vi "Measurement UI.vi"() -> ()   [LabVIEW 2021, in "audio_intermodulationDistortionMeasurement.lvlib"]
uses:
  audio_intermodulationDistortionMeasurement.lvlib
panel:
  in  "Meas Graph":T1(tab)
  out "FreqDomainGraph":cluster{"x0":dbl, "dx":dbl, "magnitude":dbl[]}(graph) caption="AC"
  out "TimeDomainGraph":waveform(dbl)(graph) caption="AC"
  out "IMD":dbl
  out "f0":dbl
  out "df":dbl
  out "Freq Domain":dbl[](array[numeric])
  out "dt":dbl
  out "Time Domain":dbl[](array[numeric])
  in  "Analog Source Resource Name":string
  out "Meas Table":string[][](table)
  out "Calculated sample rate":dbl caption="SAMPLE RATE" format="%#_6pHz"
  in  "Custom High Frequency":dbl=15000.0 caption="CUSTOM HIGH FREQUENCY" format="%_2pHz"
  in  "Custom Low Frequency":dbl=14000.0 caption="CUSTOM LOW FREQUENCY" format="%#_2pHz"
  in  "MeasSettingsOptions":i32(listbox)=-1
  in  "MeasSettings":bool
  in  "Protocol settings":string="Protocol settings"
  in  "Measurement Settings":string="Analog source "
  in  "Bit Clock Rate":u32=12288000 caption="CLOCK RATE" format="%.4pHz"
  in  "Input range":dbl=2.825 caption="INPUT RANGE" format="%#_gV"
  in  "Data Latch at SCK Cycle":u8 caption="LATCH DELAY" format="%.0fs"
  in  "Number of Words":i32=19200 caption="NUMBER OF WORDS"
  in  "Protocol Source Resource Name":string="7821\\PCMi 0" caption="RESOURCE NAME"
  in  "Amplitude":dbl=-1.0 caption="AMPLITUDE" format="%#_gdB"
  in  "IMD Standard":T2(ring) caption="IMD STANDARD"
  in  "DSGResourceName":tag="PXI1Slot3/ao0" caption="RESOURCE NAME"
  in  "Custom Amplitude Ratio":dbl=1.0 caption="CUSTOM AMPLITUDE RATIO" format="%.1f"
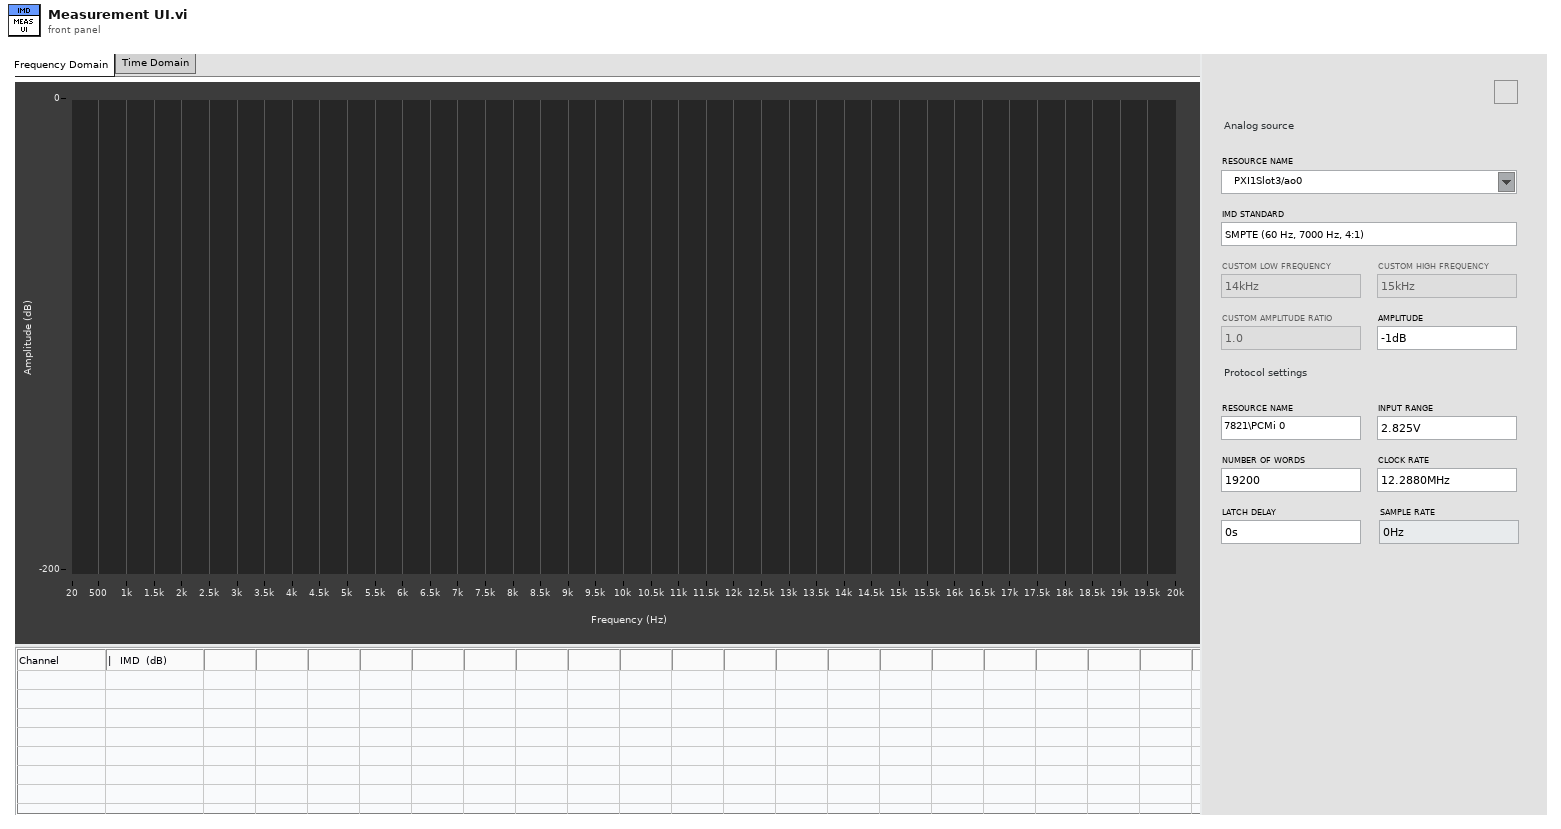
[diagram p1: front panel]
types:
  T1 = enum32{"Frequency Domain", "Time Domain", "Hidden"}
  T2 = enum16{"SMPTE (60 Hz, 7000 Hz, 4:1)", "DIN (250 Hz, 8000 Hz, 4:1)", "CCIF (11 kHz, 12 kHz, 1:1)", "CCIF (19 kHz, 20 kHz, 1:1)", "Custom"}
  T3 = enum16{"open", "replace", "create", "open or create", "replace or create", "replace or create with confirmation"}
  T4 = enum8{"Enabled", "Disabled", "Disabled and Grayed Out"}
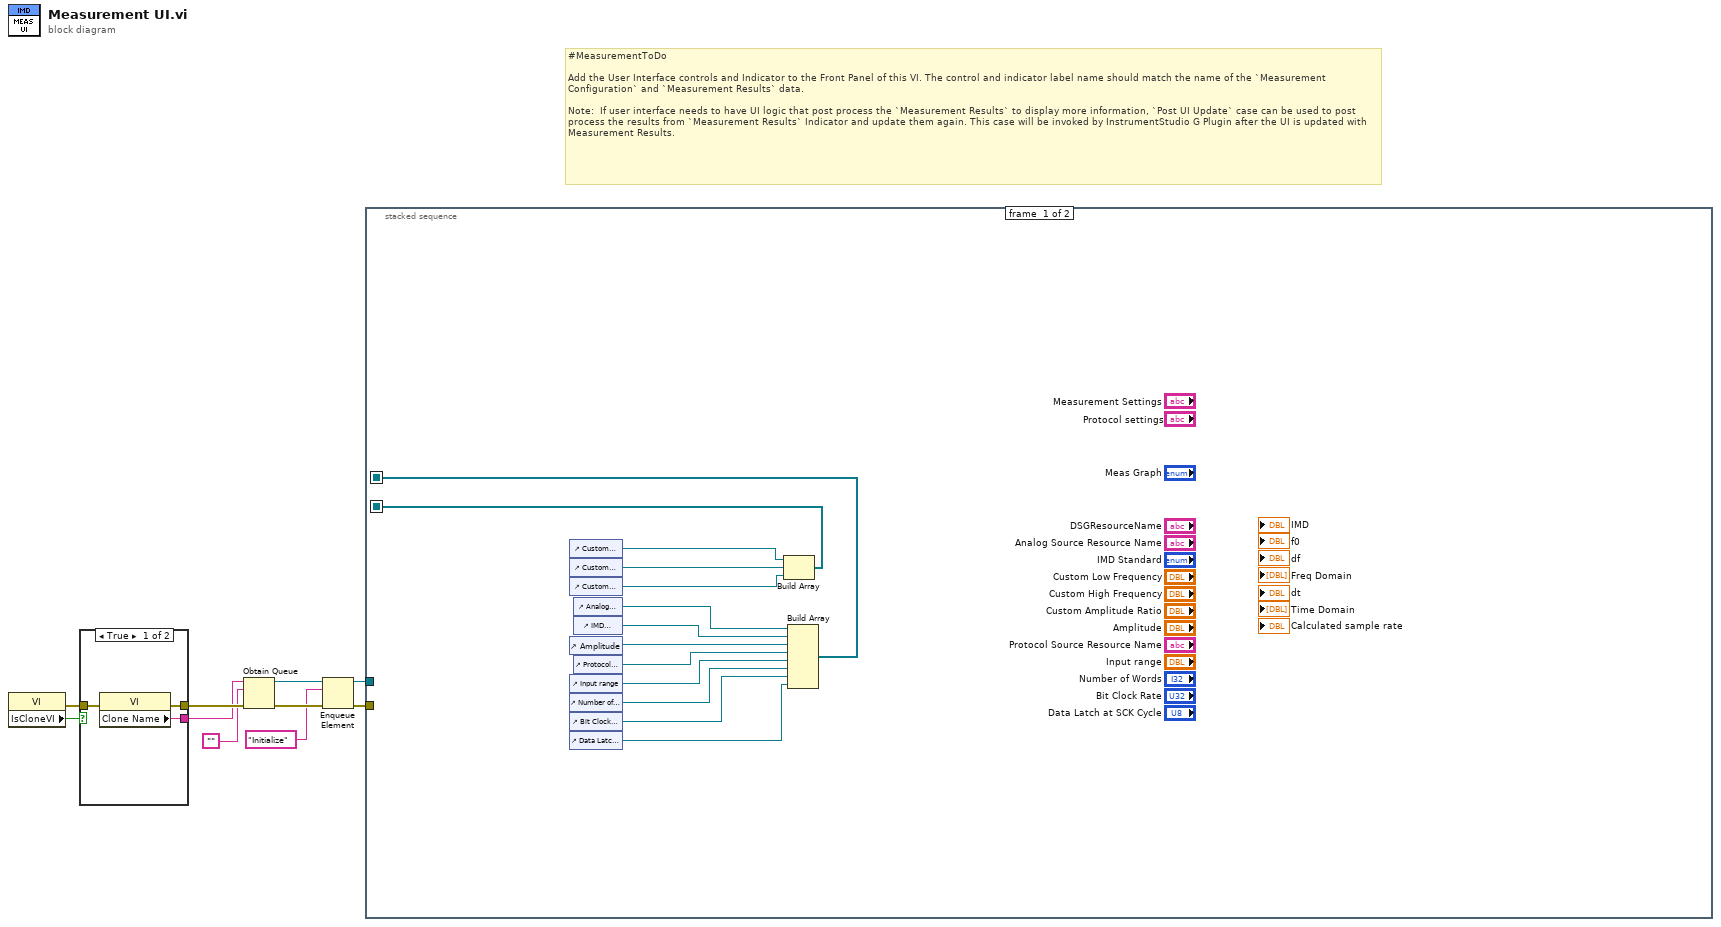
[diagram p0: block diagram]
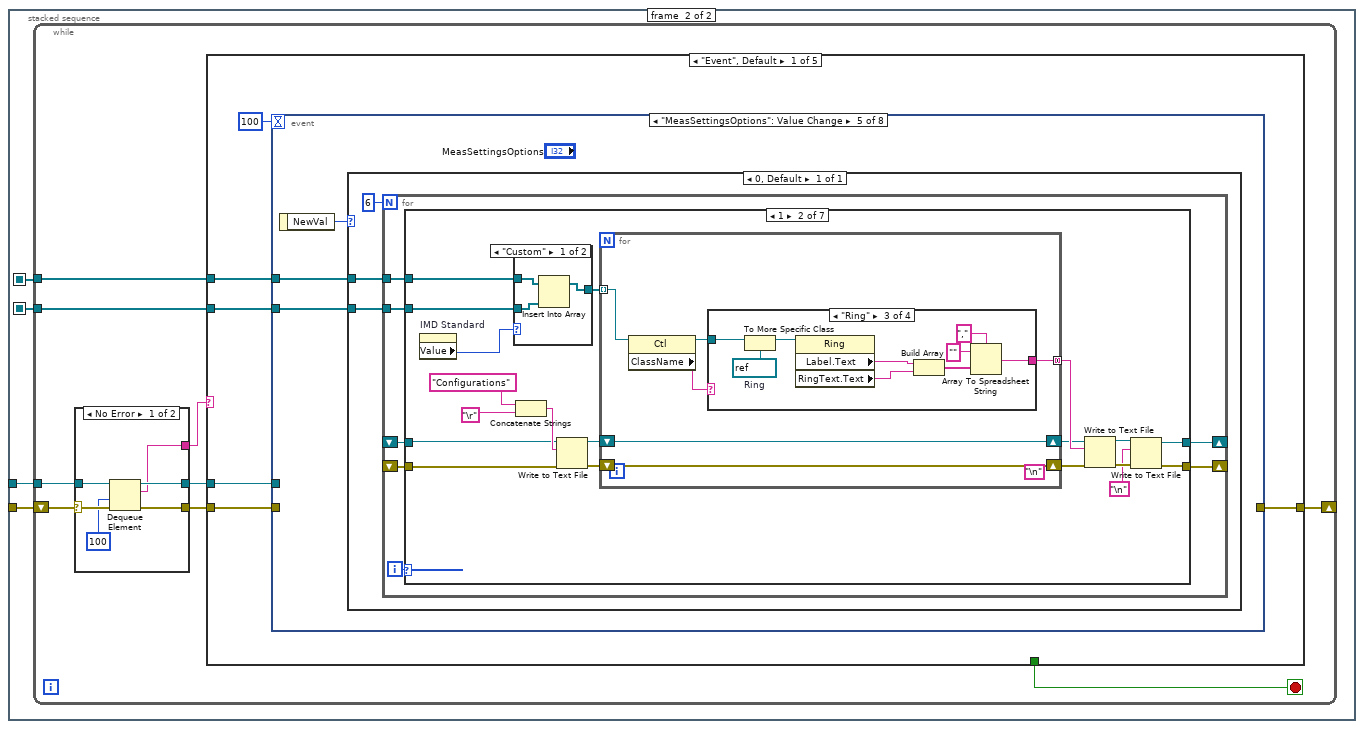
[diagram p2: hidden frame]
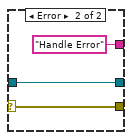
[diagram p3: hidden frame]
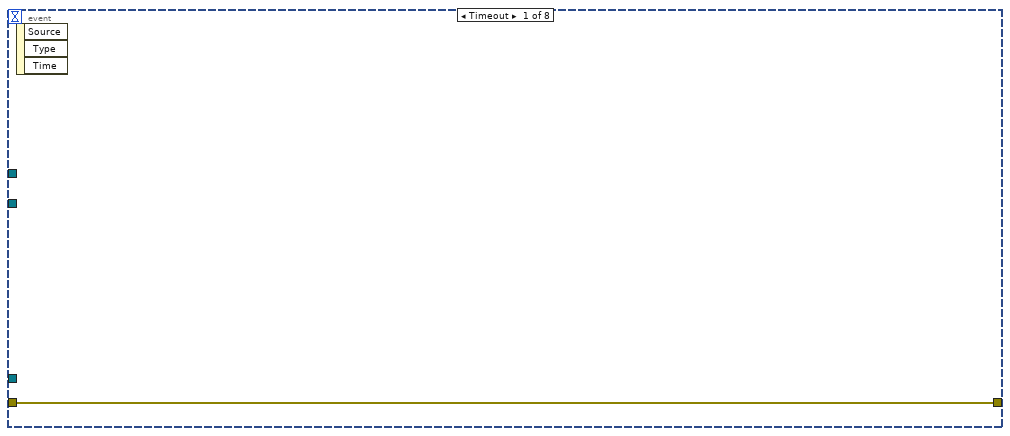
[diagram p4: hidden frame]
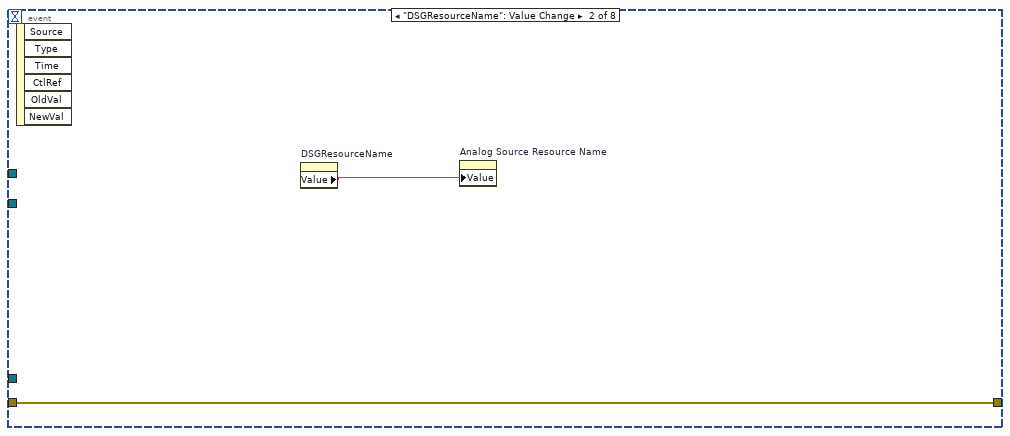
[diagram p5: hidden frame]
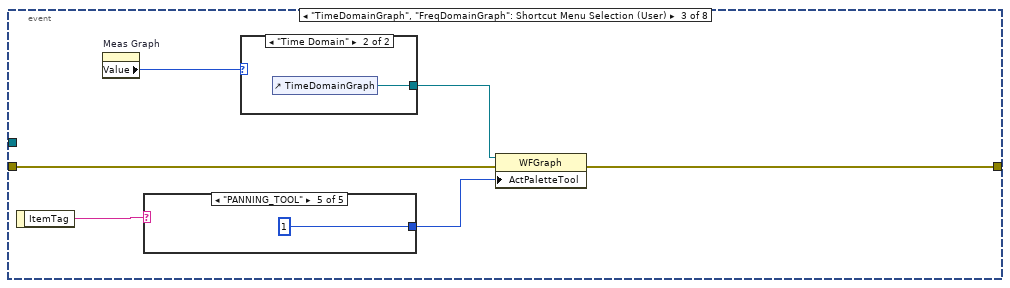
[diagram p6: hidden frame]
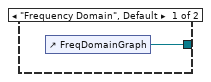
[diagram p7: hidden frame]
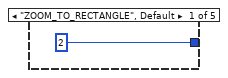
[diagram p8: hidden frame]
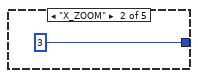
[diagram p9: hidden frame]
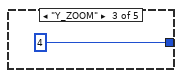
[diagram p10: hidden frame]
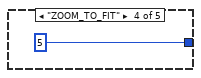
[diagram p11: hidden frame]
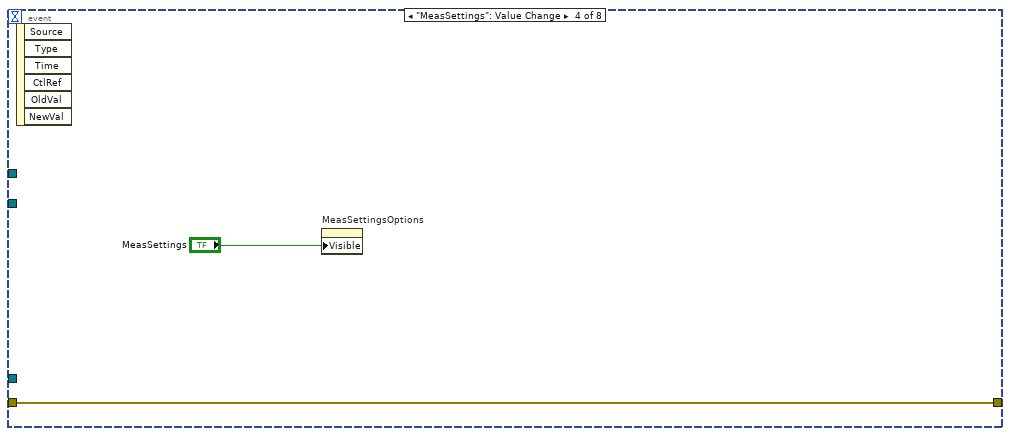
[diagram p12: hidden frame]
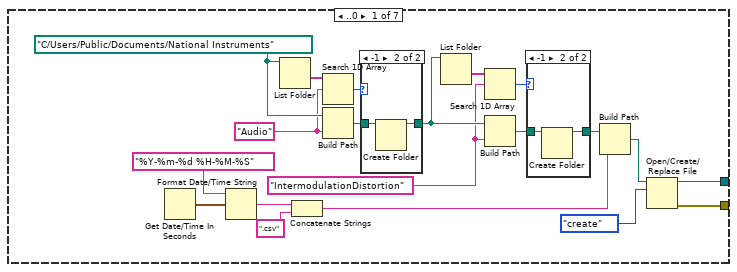
[diagram p13: hidden frame]
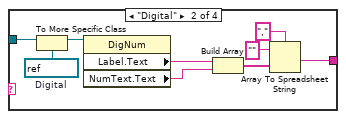
[diagram p18: hidden frame]
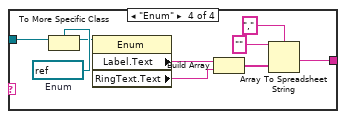
[diagram p19: hidden frame]
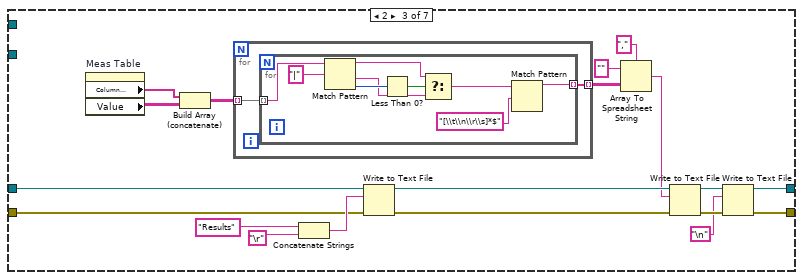
[diagram p20: hidden frame]
diagram:
  # "#MeasurementToDo  \n\nAdd the User Interface controls and Indicator to the Front Panel of this VI. The control and indicator label name should match the name of the `Measurement Configuration` and `Measurement Results` data.\n\nNote:  If user interface needs to have UI logic that post process the `Measurement Results` to display more information, `Post UI Update` case can be used to post process the results from `Measurement Results` Indicator and update them again. This case will be invoked by InstrumentStudio G Plugin after the UI is updated with Measurement Results."
  n1 = property class="VI"() -> (error out=w1:errorcluster, "IsCloneVI"=w2:bool)  [unwired: 2 in, 1 out]
  n2 = case shown="True" w2 {
    tunnel: [w13 w16] -> w10
    tunnel: [w12 w15] -> w9
    tunnel: w1 -> [w11 w14]
    frame True {
      n3 = property class="VI"(error in=w11) -> (error out=w13:errorcluster, "Clone Name"=w12:string)  [unwired: 1 in, 1 out]
    }
    frame False {
      n4 = property class="VI"(error in=w14) -> (error out=w16:errorcluster, "Name"=w15:string)  [unwired: 1 in, 1 out]
    }
  }
  n5 = Obtain Queue(name (unnamed)=w9, element data type="", error in (no error)=w10) -> (queue out=w6:refnum<queue>, error out=w8:errorcluster)  [unwired: 2 in, 1 out]
  n6 = Enqueue Element(queue=w6, element="Initialize", error in (no error)=w8) -> (queue out=w5:refnum<queue>, error out=w7:errorcluster)  [unwired: 1 in, 1 out]
  n7 = stacked-sequence {
    seq-local: [w18 _] -> [_ w30]
    seq-local: [w19 _] -> [_ w31]
    tunnel: w7 -> [_ w33]
    tunnel: w5 -> [_ w32]
    frame #0 {
      n8 = control-ref of="Custom Low Frequency"() -> (w28:refnum<vi>)
      n9 = control-ref of="Custom High Frequency"() -> (w17:refnum<vi>)
      n10 = control-ref of="Custom Amplitude Ratio"() -> (w29:refnum<vi>)
      n11 = control-ref of="Amplitude"() -> (w22:refnum<vi>)
      n12 = control-ref of="Input range"() -> (w24:refnum<vi>)
      n13 = control-ref of="Number of Words"() -> (w25:refnum<vi>)
      n14 = control-ref of="Bit Clock Rate"() -> (w26:refnum<vi>)
      n15 = control-ref of="Data Latch at SCK Cycle"() -> (w27:refnum<vi>)
      n16 = control-ref of="Analog Source Resource Name"() -> (w20:refnum<vi>)
      n17 = control-ref of="IMD Standard"() -> (w21:refnum<vi>)
      n18 = control-ref of="Protocol Source Resource Name"() -> (w23:refnum<vi>)
      n19 = Build Array(w28, w17, w29) -> (w18:refnum<vi>[])
      n20 = Build Array(w20, w21, w22, w23, w24, w25, w26, w27) -> (w19:refnum<vi>[])
    }
    frame #1 {
      n21 = while {
        shift-right: [w37] -> _
        shift-left: w33 -> [w42]
        tunnel: w32 -> [w40]
        tunnel: w30 -> [w35]
        tunnel: w31 -> [w34]
        stop <- w36 stop-if-true
        n22 = case shown="No Error" w42 {
          selector: w42 -> [w48 w51]
          tunnel: [w47 w51] -> w41
          tunnel: w40 -> [w46 w50]
          tunnel: [w45 w50] -> w39
          tunnel: [w44 "Handle Error"] -> w38
          frame No Error {
            n23 = Dequeue Element(queue=w46, timeout in ms (-1)=100, error in (no error)=w48) -> (queue out=w45:refnum<queue>, element=w44:string, error out=w47:errorcluster)  [unwired: 1 out]
          }
          frame Error {
          }
        }
        n24 = case shown="\"Event\", Default" w38 {
          tunnel: w41 -> [w56 w297 w322 w329 w330]
          tunnel: w39 -> [w54 _ _ w327 _]
          tunnel: [w57 w297 w322 w324 w330] -> w37
          tunnel: [_ FALSE _ TRUE _] -> w36
          tunnel: w35 -> [w53 _ _ _ _]
          tunnel: w34 -> [w52 _ _ _ _]
          frame "Event", Default {
            n25 = event shown="[4] \"MeasSettingsOptions\": Value Change" {
              selector: _ -> [_ _ _ _ _ _ _ _]
              dyn-events: _ -> [_ _ _ _ _ _ _ _]
              timeout: 100 -> [_ _ _ _ _ _ _ _]
              tunnel: [w58 w59 w65 w74 _ _ _ w285] -> w57
              tunnel: w56 -> [w58 w59 w66 w74 _ _ _ w286]
              tunnel: w54 -> [_ _ _ _ _ _ _ w284]
              tunnel: w53 -> [_ _ _ _ w77 _ _ _]
              tunnel: w52 -> [_ _ _ _ w76 _ _ _]
              event Timeout {
                n26 = event-data() -> ()  [unwired: 1 in, 3 out]
              }
              event "DSGResourceName": Value Change {
                n27 = event-data() -> ()  [unwired: 1 in, 6 out]
                n28 = property on="DSGResourceName" class="DAQmxName"() -> ("Value"=w60:string)  [unwired: 2 in, 2 out]
                n29 = property on="Analog Source Resource Name" class="Str"("Value"=w60) -> ()  [unwired: 2 in, 2 out]
              }
              event "TimeDomainGraph", "FreqDomainGraph": Shortcut Menu Selection (User) {
                n30 = event-data() -> ("ItemTag"=w64:string)  [unwired: 1 in]
                n31 = property on="Meas Graph" class="TabCtl (strict)"() -> ("Value"=w62:T1)  [unwired: 2 in, 2 out]
                n32 = case shown="\"PANNING_TOOL\"" w64 {
                  tunnel: [2 3 4 5 1] -> w63
                  frame "ZOOM_TO_RECTANGLE", Default {
                  }
                  frame "X_ZOOM" {
                  }
                  frame "Y_ZOOM" {
                  }
                  frame "ZOOM_TO_FIT" {
                  }
                  frame "PANNING_TOOL" {
                  }
                }
                n33 = case shown="\"Time Domain\"" w62 {
                  tunnel: [w67 w68] -> w61
                  frame "Frequency Domain", Default {
                    n34 = control-ref of="FreqDomainGraph"() -> (w67:refnum<vi>)
                  }
                  frame "Time Domain" {
                    n35 = control-ref of="TimeDomainGraph"() -> (w68:refnum<vi>)
                  }
                }
                n36 = property class="WFGraph"(reference=w61, error in=w66, "ActPaletteTool"=w63) -> (error out=w65:errorcluster)  [unwired: 1 out]
              }
              event "MeasSettings": Value Change {
                n37 = event-data() -> ()  [unwired: 1 in, 6 out]
                n38 = property on="MeasSettingsOptions" class="LstBox (strict)"("Visible"="MeasSettings") -> ()  [unwired: 2 in, 2 out]
              }
              event "MeasSettingsOptions": Value Change {
                n39 = event-data() -> ("NewVal"=w78:i32)  [unwired: 1 in]
                n40 = case shown="0, Default" w78 {
                  tunnel: w77 -> [w80]
                  tunnel: w76 -> [w79]
                  frame 0, Default {
                    n41 = for {
                      N: 6 -> [_]
                      shift-right: [w87] -> _
                      shift-left: _ -> [w85]
                      shift-right: [w86] -> _
                      shift-left: _ -> [w84]
                      tunnel: w80 -> [w83]
                      tunnel: w79 -> [w82]
                      i -> [w88]
                      n42 = case shown="1" w88 {
                        tunnel: [w90 w121 w175 w205 w242 refnum<file> refnum ("refnum out") w275] -> w87
                        tunnel: [w89 w122 w176 w206 w241 w270 w276] -> w86
                        tunnel: w85 -> [_ w120 w174 w203 w239 w272 w275]
                        tunnel: w84 -> [_ w119 w173 w204 w240 w271 w276]
                        tunnel: w83 -> [_ w116 _ _ _ _ _]
                        tunnel: w82 -> [_ w117 _ _ _ _ _]
                        frame ..0 {
                          w99 = "IntermodulationDistortion" ("prompt")
                          w104 = "Audio" ("prompt")
                          w107 = path "C:/Users/Public/Documents/National Instruments" ("base path")
                          n43 = Get Date/Time In Seconds() -> (seconds since 1Jan1904=w96:timestamp)
                          n44 = Format Date/Time String(time format string (%c)="%Y-%m-%d %H-%M-%S", seconds (now)=w96) -> (date/time string=w95:string)  [unwired: 1 in]
                          n45 = List Folder(path=w107) -> (folder names=w105:string[])  [unwired: 3 in, 3 out]
                          n46 = Concatenate Strings(w95, ".csv" ("string")) -> (w92:string)
                          n47 = Search 1D Array(1D array=w105, element=w104) -> (index of element=w103:i32)  [unwired: 1 in]
                          n48 = Build Path(base path=w107, name or relative path=w104) -> (appended path=w106:path)
                          n49 = case shown="-1" w103 {
                            tunnel: w106 -> [w112 w114]
                            tunnel: [w112 w113] -> w100
                            frame Default {
                            }
                            frame -1 {
                              n50 = Create Folder(path (use dialog)=w114) -> (created path=w113:path)  [unwired: 2 in, 2 out]
                            }
                          }
                          n51 = List Folder(path=w100) -> (folder names=w102:string[])  [unwired: 3 in, 3 out]
                          n52 = Search 1D Array(1D array=w102, element=w99) -> (index of element=w101:i32)  [unwired: 1 in]
                          n53 = Build Path(base path=w100, name or relative path=w99) -> (appended path=w98:path)
                          n54 = case shown="-1" w101 {
                            tunnel: w98 -> [w109 w111]
                            tunnel: [w109 w110] -> w93
                            frame Default {
                            }
                            frame -1 {
                              n55 = Create Folder(path (use dialog)=w111) -> (created path=w110:path)  [unwired: 2 in, 2 out]
                            }
                          }
                          n56 = Build Path(base path=w93, name or relative path=w92) -> (appended path=w91:path)
                          n57 = Open/Create/Replace File(file path (use dialog)=w91, operation (0:open)=T3."create") -> (refnum out=w90:refnum<file>, error out=w89:errorcluster)  [unwired: 4 in, 1 out]
                        }
                        frame 1 {
                          (unwired) "\n"
                          n58 = property on="IMD Standard" class="Enum (strict)"() -> ("Value"=w118:T2)  [unwired: 2 in, 2 out]
                          n59 = case shown="\"Custom\"" w118 {
                            tunnel: w117 -> [w135 w137]
                            tunnel: w116 -> [w134 _]
                            tunnel: [w136 w137] -> w115
                            frame "Custom" {
                              n60 = Insert Into Array(array=w135, new element=w134) -> (w136:refnum<vi>[])  [unwired: 1 in]
                            }
                            frame Default {
                            }
                          }
                          n61 = Concatenate Strings("Configurations" ("format string"), "\r") -> (w131:string)
                          n62 = Write to Text File(file (use dialog)=w120, text=w131, error in=w119) -> (refnum out=w129:refnum<file>, error out=w130:errorcluster)  [unwired: 1 in, 1 out]
                          n63 = for {
                            shift-right: [w143] -> w127
                            shift-left: w129 -> [w143]
                            shift-right: [w142] -> w126
                            shift-left: w130 -> [w142]
                            tunnel: [w141] -> w128 mode=concatenating
                            tunnel: w115 -> [w138] mode=indexing
                            n64 = property class="Ctl"(reference=w138) -> (reference out=w140:refnum<vi>, "ClassName"=w139:string)  [unwired: 1 in, 1 out]
                            n65 = case shown="\"Ring\"" w139 {
                              tunnel: [_ w147 w157 w166] -> w141
                              tunnel: w140 -> [_ w145 w155 w170]
                              frame Default {
                              }
                              frame "Digital" {
                                w144 = refnum<vi> refnum  # Digital
                                n66 = To More Specific Class(target class=w144, reference=w145) -> (specific class reference=w146:refnum<vi>)  [unwired: 1 in, 1 out]
                                n67 = property class="DigNum"(reference=w146) -> ("Label.Text"=w152:string, "NumText.Text"=w151:string)  [unwired: 1 in, 2 out]
                                n68 = Build Array(w152, w151) -> (w148:string[])
                                n69 = Array To Spreadsheet String(delimiter (Tab)=",", array=w148, 3:"" ("format string")) -> (spreadsheet string=w147:string)
                              }
                              frame "Ring" {
                                w154 = refnum<vi> refnum  # Ring
                                n70 = To More Specific Class(target class=w154, reference=w155) -> (specific class reference=w156:refnum<vi>)  [unwired: 1 in, 1 out]
                                n71 = property class="Ring"(reference=w156) -> ("Label.Text"=w153:string, "RingText.Text"=w161:string)  [unwired: 1 in, 2 out]
                                n72 = Build Array(w153, w161) -> (w158:string[])
                                n73 = Array To Spreadsheet String(delimiter (Tab)=",", array=w158, 3:"" ("format string")) -> (spreadsheet string=w157:string)
                              }
                              frame "Enum" {
                                w169 = refnum<vi> refnum  # Enum
                                n74 = To More Specific Class(target class=w169, reference=w170) -> (specific class reference=w165:refnum<vi>)  [unwired: 1 in, 1 out]
                                n75 = property class="Enum"(reference=w165) -> ("Label.Text"=w164:string, "RingText.Text"=w163:string)  [unwired: 1 in, 2 out]
                                n76 = Build Array(w164, w163) -> (w162:string[])
                                n77 = Array To Spreadsheet String(delimiter (Tab)=",", array=w162, 3:"" ("format string")) -> (spreadsheet string=w166:string)
                              }
                            }
                          }
                          n78 = Write to Text File(file (use dialog)=w127, text=w128, error in=w126) -> (refnum out=w125:refnum<file>, error out=w124:errorcluster)  [unwired: 1 in, 1 out]
                          n79 = Write to Text File(file (use dialog)=w125, text="\n", error in=w124) -> (refnum out=w121:refnum<file>, error out=w122:errorcluster)  [unwired: 1 in, 1 out]
                        }
                        frame 2 {
                          n80 = property on="Meas Table" class="Tbl (strict)"() -> ("Column Headers[]"=w171:string[], "Value"=w172:string[][])  [unwired: 2 in, 2 out]
                          n81 = Build Array (concatenate)(w171, w172) -> (w188:string[][])
                          n82 = for {
                            tunnel: w188 -> [w191] mode=indexing
                            tunnel: [w190] -> w187 mode=indexing
                            n83 = for {
                              tunnel: w191 -> [w193] mode=indexing
                              tunnel: [w192] -> w190 mode=indexing
                              n84 = Match Pattern(string=w193, regular expression="|") -> (before substring=w197:string, after substring=w196:string, offset past match=w199:i32)  [unwired: 1 in, 1 out]
                              n85 = Less Than 0?(x=w199) -> (x < 0?=w198:bool)
                              n86 = Select(t=w197, s=w198, f=w196) -> (s? t:f=w195:string)
                              n87 = Match Pattern(string=w195, regular expression="[\\t\\n\\r\\s]*$") -> (before substring=w192:string)  [unwired: 1 in, 3 out]
                            }
                          }
                          n88 = Concatenate Strings("Results" ("element"), "\r") -> (w177:string)
                          n89 = Write to Text File(file (use dialog)=w174, text=w177, error in=w173) -> (refnum out=w189:refnum<file>, error out=w183:errorcluster)  [unwired: 1 in, 1 out]
                          n90 = Array To Spreadsheet String(delimiter (Tab)=",", array=w187, 3:"" ("format string")) -> (spreadsheet string=w184:string)
                          n91 = Write to Text File(file (use dialog)=w189, text=w184, error in=w183) -> (refnum out=w182:refnum<file>, error out=w181:errorcluster)  [unwired: 1 in, 1 out]
                          n92 = Write to Text File(file (use dialog)=w182, text="\n", error in=w181) -> (refnum out=w175:refnum<file>, error out=w176:errorcluster)  [unwired: 1 in, 1 out]
                        }
                        frame 3 {
                          n93 = property on="FreqDomainGraph" class="WFGraph (strict)"() -> ("Value"=w201:cluster{"x0":dbl, "dx":dbl, "magnitude":dbl[]})  [unwired: 2 in, 2 out]
                          n94 = Concatenate Strings("Frequency Domain" ("string"), "\r") -> (w228:string)
                          n95 = Build Array("Frequency (Hz)", "Amplitude (dB)") -> (w227:string[])
                          n96 = Write to Text File(file (use dialog)=w203, text=w228, error in=w204) -> (refnum out=w224:refnum<file>, error out=w223:errorcluster)  [unwired: 1 in, 1 out]
                          n97 = Unbundle By Name(w201) -> ("dx"=w215:dbl, "x0"=w216:dbl, "magnitude"=w214:dbl[])
                          n98 = Array To Spreadsheet String(delimiter (Tab)=",", array=w227, 3:"" ("format string")) -> (spreadsheet string=w222:string)
                          n99 = Write to Text File(file (use dialog)=w224, text=w222, error in=w223) -> (refnum out=w221:refnum<file>, error out=w220:errorcluster)  [unwired: 1 in, 1 out]
                          n100 = for {
                            tunnel: w214 -> [w232] mode=indexing
                            tunnel: w215 -> [w236]
                            tunnel: w216 -> [w234]
                            tunnel: [w229] -> w217 mode=indexing
                            i -> [w237]
                            n101 = Multiply(x=w237, y=w236) -> (x*y=w235:dbl)
                            n102 = Add(x=w235, y=w234) -> (x+y=w233:dbl)
                            n103 = Format Into String(w233) -> (resulting string=w230:string)  [unwired: 3 in, 1 out]
                            n104 = Format Into String(w232) -> (resulting string=w231:string)  [unwired: 3 in, 1 out]
                            n105 = Build Array(w230, w231) -> (w229:string[])
                          }
                          n106 = Array To Spreadsheet String(delimiter (Tab)=",", array=w217, 3:"" ("format string")) -> (spreadsheet string=w213:string)
                          n107 = Write to Text File(file (use dialog)=w221, text=w213, error in=w220) -> (refnum out=w211:refnum<file>, error out=w210:errorcluster)  [unwired: 1 in, 1 out]
                          n108 = Write to Text File(file (use dialog)=w211, text="\n", error in=w210) -> (refnum out=w205:refnum<file>, error out=w206:errorcluster)  [unwired: 1 in, 1 out]
                        }
                        frame 4 {
                          n109 = property on="TimeDomainGraph" class="WFGraph (strict)"() -> ("Value"=w238:waveform(dbl))  [unwired: 2 in, 2 out]
                          n110 = Concatenate Strings("Time Domain" ("string"), "\r") -> (w260:string)
                          n111 = Write to Text File(file (use dialog)=w239, text=w260, error in=w240) -> (refnum out=w257:refnum<file>, error out=w256:errorcluster)  [unwired: 1 in, 1 out]
                          n112 = Build Array("Time (s)", "Amplitude (V)") -> (w259:string[])
                          n113 = Unbundle By Name(w238) -> ("dt"=w247:dbl, "Y"=w248:dbl[])
                          n114 = Array To Spreadsheet String(delimiter (Tab)=",", array=w259, 3:"" ("format string")) -> (spreadsheet string=w255:string)
                          n115 = Write to Text File(file (use dialog)=w257, text=w255, error in=w256) -> (refnum out=w254:refnum<file>, error out=w253:errorcluster)  [unwired: 1 in, 1 out]
                          n116 = for {
                            tunnel: [w266] -> w250 mode=indexing
                            tunnel: w248 -> [w265] mode=indexing
                            tunnel: w247 -> [w263]
                            i -> [w264]
                            n117 = Multiply(x=w263, y=w264) -> (x*y=w262:dbl)
                            n118 = Format Into String(w262) -> (resulting string=w267:string)  [unwired: 3 in, 1 out]
                            n119 = Format Into String(w265) -> (resulting string=w268:string)  [unwired: 3 in, 1 out]
                            n120 = Build Array(w267, w268) -> (w266:string[])
                          }
                          n121 = Array To Spreadsheet String(delimiter (Tab)=",", array=w250, 3:"" ("format string")) -> (spreadsheet string=w249:string)
                          n122 = Write to Text File(file (use dialog)=w254, text=w249, error in=w253) -> (refnum out=w242:refnum<file>, error out=w241:errorcluster)  [unwired: 1 in, 1 out]
                        }
                        frame 5 {
                          w273 = FALSE ("Visible")
                          n123 = Close File(refnum=w272, error in=w271) -> (error out=w270:errorcluster)  [unwired: 1 out]
                          n124 = property on="MeasSettingsOptions" class="LstBox (strict)"("Visible"=w273, "Value"=-1 ("MeasSettingsOptions")) -> ()  [unwired: 2 in, 2 out]
                          n125 = property on="MeasSettings" class="Bool (strict)"("Value"=w273) -> ()  [unwired: 2 in, 2 out]
                        }
                        frame Default {
                        }
                      }
                    }
                  }
                }
              }
              event Mouse Down {
                w277 = FALSE ("Visible")
                n126 = event-data() -> ()  [unwired: 1 in, 1 out]
                n127 = property on="MeasSettingsOptions" class="LstBox (strict)"("Visible"=w277, "Value"=-1 ("MeasSettingsOptions")) -> ()  [unwired: 2 in, 2 out]
                n128 = property on="MeasSettings" class="Bool (strict)"("Value"=w277) -> ()  [unwired: 2 in, 2 out]
              }
              event "IMD Standard": Value Change {
                n129 = event-data() -> ()  [unwired: 1 in, 6 out]
                n130 = local read "IMD Standard"() -> (w280:T2)
                n131 = case shown="Default" w280 {
                  tunnel: [T4."Enabled" ("Disabled") T4."Disabled and Grayed Out" ("Disabled")] -> w279
                  frame "Custom" {
                  }
                  frame Default {
                  }
                }
                n132 = property on="Custom Low Frequency" class="DigNum (strict)"("DisabledEnum"=w279) -> ()  [unwired: 2 in, 2 out]
                n133 = property on="Custom High Frequency" class="DigNum (strict)"("DisabledEnum"=w279) -> ()  [unwired: 2 in, 2 out]
                n134 = property on="Custom Amplitude Ratio" class="DigNum (strict)"("DisabledEnum"=w279) -> ()  [unwired: 2 in, 2 out]
              }
              event Panel Close? {
                n135 = event-data() -> ()  [unwired: 1 in, 4 out]
                n136 = Enqueue Element(queue=w284, element="Exit", error in (no error)=w286) -> (error out=w285:errorcluster)  [unwired: 1 in, 2 out]
                n137 = event-data("Discard?"=TRUE) -> ()  [unwired: 1 in, 1 out]
              }
            }
          }
          frame "Initialize" {
            w290 = string[] ["Export data"] ("Item Names")
            n138 = local read "IMD Standard"() -> (w289:T2)
            n139 = case shown="Default" w289 {
              tunnel: [T4."Enabled" ("Disabled") T4."Disabled and Grayed Out" ("Disabled")] -> w288
              frame "Custom" {
              }
              frame Default {
              }
            }
            n140 = property on="DSGResourceName" class="DAQmxName"("Value"="<Select Device>") -> ()  [unwired: 2 in, 2 out]
            n141 = property on="Custom Low Frequency" class="DigNum (strict)"("DisabledEnum"=w288) -> ()  [unwired: 2 in, 2 out]
            n142 = property on="Custom High Frequency" class="DigNum (strict)"("DisabledEnum"=w288) -> ()  [unwired: 2 in, 2 out]
            n143 = property on="Custom Amplitude Ratio" class="DigNum (strict)"("DisabledEnum"=w288) -> ()  [unwired: 2 in, 2 out]
            n144 = for {
              N: 2 -> [_]
              i -> [w304]
              n145 = case shown="0, Default" w304 {
                tunnel: [w305 w306] -> w303
                frame 0, Default {
                  n146 = control-ref of="FreqDomainGraph"() -> (w305:refnum<vi>)
                }
                frame 1 {
                  n147 = control-ref of="TimeDomainGraph"() -> (w306:refnum<vi>)
                }
              }
              n148 = property class="WFGraph"(reference=w303, "ActPaletteTool"=2 ("Palette:Active Tool")) -> ()  [unwired: 1 in, 2 out]
            }
            n149 = property on="MeasSettingsOptions" class="LstBox (strict)"("Item Names"=w290, "Value"=-1 ("MeasSettingsOptions"), "Visible"=FALSE, "Disabled Items"=i32[] []) -> ()  [unwired: 2 in, 2 out]
            n150 = for {
              tunnel: w290 -> [_] mode=indexing
              i -> [w301]
              n151 = property on="MeasSettingsOptions" class="LstBox (strict)"("Active Row"=w301, "Cell Height"=30 ("Active Row:Cell Height")) -> ()  [unwired: 2 in, 2 out]
            }
          }
          frame "Post UI Update" {
            # "This case will be triggered, after framework updates the User interface with result values."
            n152 = local read "IMD"() -> (w313:dbl)
            n153 = local read "Freq Domain"() -> (w319:dbl[])
            n154 = local read "df"() -> (w318:dbl)
            n155 = local read "f0"() -> (w317:dbl)
            n156 = local read "Time Domain"() -> (w315:dbl[])
            n157 = local read "dt"() -> (w314:dbl)
            n158 = local read "Protocol Source Resource Name"() -> (w310:string)
            n159 = Format Into String(format string="%5.1f", initial string="|   ", w313) -> (resulting string=w309:string)  [unwired: 1 in, 1 out]
            n160 = Bundle By Name(cluster=cluster{"x0":dbl, "dx":dbl, "magnitude":dbl[]} {"x0"=0.0, "dx"=0.0, "magnitude"=[]} ("FreqDomainGraph"), "x0"=w317, "dx"=w318, "magnitude"=w319) -> (→"FreqDomainGraph":cluster{"x0":dbl, "dx":dbl, "magnitude":dbl[]})
            n161 = Build Array(w310, w309) -> (w308:string[])
            n162 = Bundle By Name("Y"=w315, "dt"=w314) -> (→"TimeDomainGraph":waveform(dbl))  [unwired: 1 in]
            n163 = Build Array(w308) -> (→"Meas Table":string[][])
          }
          frame "Exit" {
            # "This case is triggered to close the User Interface from framework"
            n164 = Flush Queue(queue=w327, error in (no error)=w329) -> (queue out=w326:refnum<queue>, error out=w325:errorcluster)  [unwired: 1 out]
            n165 = Release Queue(queue=w326, force destroy? (F)=TRUE, error in (no error)=w325) -> (error out=w324:errorcluster)  [unwired: 2 out]
          }
          frame "Handle Error" {
          }
        }
      }
    }
  }
